vi "Calculo_conversao.vi"(8 "Tipo":enum16{"Saida", "Entrada"}(ring), 9 "Min":dbl, 10 "Max":dbl, 11 "Value":variant) -> (3 "Value 2":variant)   [LabVIEW 2019]
uses:
  <vilib>/Utility/Data Type/NI_Data Type.lvlib
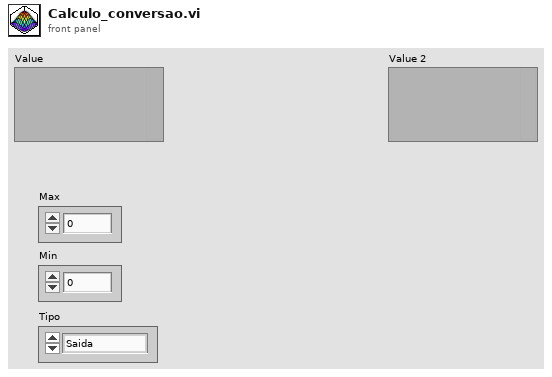
[diagram p1: front panel]
types:
  T1 = typedef "NI_Data Type.lvlib/Data Type.ctl" = enum8{"Invalid Type", "Void", "I8", "I16", "I32", "I64", "U8", "U16", "U32", "U64", "Single Float", "Double Float", "Extended Float", "Single Complex", "Double Complex", "Extended Complex", "Enum U8", "Enum U16", "Enum U32", "Enum U64", "Single Float With Unit", "Double Float With Unit", "Extended Float With Unit", "Single Complex with Unit", "Double Complex with Unit", "Extended Complex with Unit", "Boolean", "String", "Path", "Picture", "Tag", "Array", "Cluster", "Variant", "LV Variant", "Waveform", "Timestamp", "Digital Waveform", "Digital Data", "ExpressData", "Refnum", "External Data", "VI", "Poly VI", "LabVIEW Class Instance", "Fixed Point", "Set Collection", "Map Collection"}
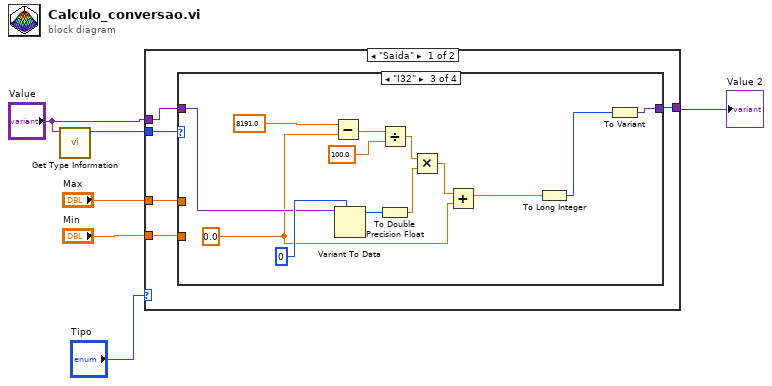
[diagram p0: block diagram]
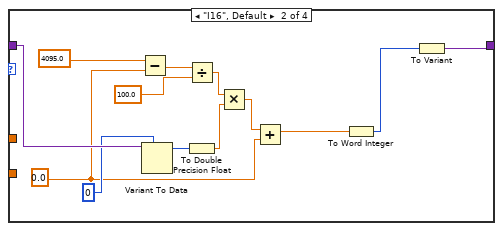
[diagram p3: hidden frame]
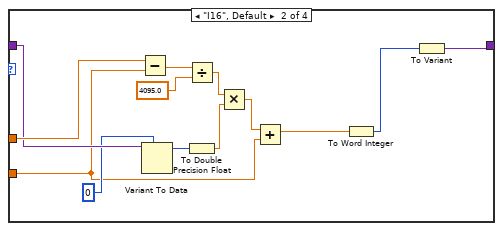
[diagram p7: hidden frame]
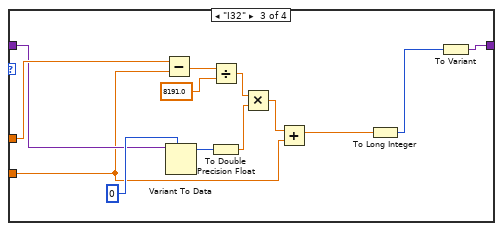
[diagram p8: hidden frame]
diagram:
  n1 = call <vilib>:"Get Type Information.vi"("variant"="Value") -> ("type"=w5:T1)  [unwired: 6 in, 4 out]
  n2 = case shown="\"Saida\"" "Tipo" {
    tunnel: "Value" -> [w10 w40]
    tunnel: w5 -> [w11 w44]
    tunnel: "Max" -> [w8 w43]
    tunnel: "Min" -> [w7 w42]
    tunnel: [w9 w41] -> w1
    frame "Saida" {
      n3 = case shown="\"I32\"" w11 {
        tunnel: [w12 w17 w28 w39] -> w9
        tunnel: w8 -> [_ _ _ _]
        tunnel: w7 -> [_ _ _ _]
        tunnel: w10 -> [w12 w23 w29 w39]
        frame "Invalid Type" {
        }
        frame "I16", Default {
          w14 = 0.0
          n4 = Subtract(x=4095.0, y=w14) -> (x-y=w25:dbl)
          n5 = Variant To Data(type=i16 0, Variant=w23) -> (data=w20:i16)  [unwired: 1 in, 1 out]
          n6 = Divide(x=w25, y=100.0) -> (x/y=w24:dbl)
          n7 = To Double Precision Float(number=w20) -> (double precision float=w21:dbl)
          n8 = Multiply(x=w24, y=w21) -> (x*y=w19:dbl)
          n9 = Add(x=w19, y=w14) -> (x+y=w18:dbl)
          n10 = To Word Integer(number=w18) -> (16bit integer=w16:i16)
          n11 = To Variant(anything=w16) -> (Variant=w17:variant)
        }
        frame "I32" {
          w26 = 0.0 ("y")
          n12 = Subtract(x=8191.0, y=w26) -> (x-y=w38:dbl)
          n13 = Variant To Data(type=i16 0, Variant=w29) -> (data=w35:i16)  [unwired: 1 in, 1 out]
          n14 = Divide(x=w38, y=100.0) -> (x/y=w37:dbl)
          n15 = To Double Precision Float(number=w35) -> (double precision float=w36:dbl)
          n16 = Multiply(x=w37, y=w36) -> (x*y=w34:dbl)
          n17 = Add(x=w34, y=w26) -> (x+y=w33:dbl)
          n18 = To Long Integer(number=w33) -> (32bit integer=w32:i32)
          n19 = To Variant(anything=w32) -> (Variant=w28:variant)
        }
        frame "Double Float" {
        }
      }
    }
    frame "Entrada", Default {
      n20 = case shown="\"Double Float\"" w44 {
        tunnel: [w45 w47 w59 w72] -> w41
        tunnel: w43 -> [_ w58 w62 _]
        tunnel: w42 -> [_ w49 w60 _]
        tunnel: w40 -> [w45 w54 w61 w72]
        frame "Invalid Type" {
        }
        frame "I16", Default {
          n21 = Subtract(x=w58, y=w49) -> (x-y=w57:dbl)
          n22 = Variant To Data(type=i16 0, Variant=w54) -> (data=w51:i16)  [unwired: 1 in, 1 out]
          n23 = Divide(x=w57, y=4095.0) -> (x/y=w55:dbl)
          n24 = To Double Precision Float(number=w51) -> (double precision float=w52:dbl)
          n25 = Multiply(x=w55, y=w52) -> (x*y=w50:dbl)
          n26 = Add(x=w50, y=w49) -> (x+y=w48:dbl)
          n27 = To Word Integer(number=w48) -> (16bit integer=w46:i16)
          n28 = To Variant(anything=w46) -> (Variant=w47:variant)
        }
        frame "I32" {
          n29 = Subtract(x=w62, y=w60) -> (x-y=w71:dbl)
          n30 = Variant To Data(type=i16 0, Variant=w61) -> (data=w68:i16)  [unwired: 1 in, 1 out]
          n31 = Divide(x=w71, y=8191.0) -> (x/y=w70:dbl)
          n32 = To Double Precision Float(number=w68) -> (double precision float=w69:dbl)
          n33 = Multiply(x=w70, y=w69) -> (x*y=w67:dbl)
          n34 = Add(x=w67, y=w60) -> (x+y=w66:dbl)
          n35 = To Long Integer(number=w66) -> (32bit integer=w65:i32)
          n36 = To Variant(anything=w65) -> (Variant=w59:variant)
        }
        frame "Double Float" {
        }
      }
    }
  }
  "Value 2" <- w1
